vi "MDB Reference.vi"(8 "error in (no error)":errorcluster, 11 "Collaudi T/motori F":bool) -> (0 "error out":errorcluster, 2 "DB rete(F) Locale(T)":bool, 3 "Refnum out":T1)   [LabVIEW 2019]
uses:
  <vilib>/addons/database/Connection.llb/Conn ObjectReference.ctl
  <vilib>/Utility/file.llb/Read From Spreadsheet File (string).vi
  <vilib>/addons/database/Connection.llb/DB Tools Open Connec (String).vi
  Global scelta DB rete o Locale.vi
  <vilib>/addons/database/Connection.llb/DB Tools Open Connec (Path).vi
  <vilib>/addons/database/NI_Database_API.lvlib
panel:
  out "Numeric":i32
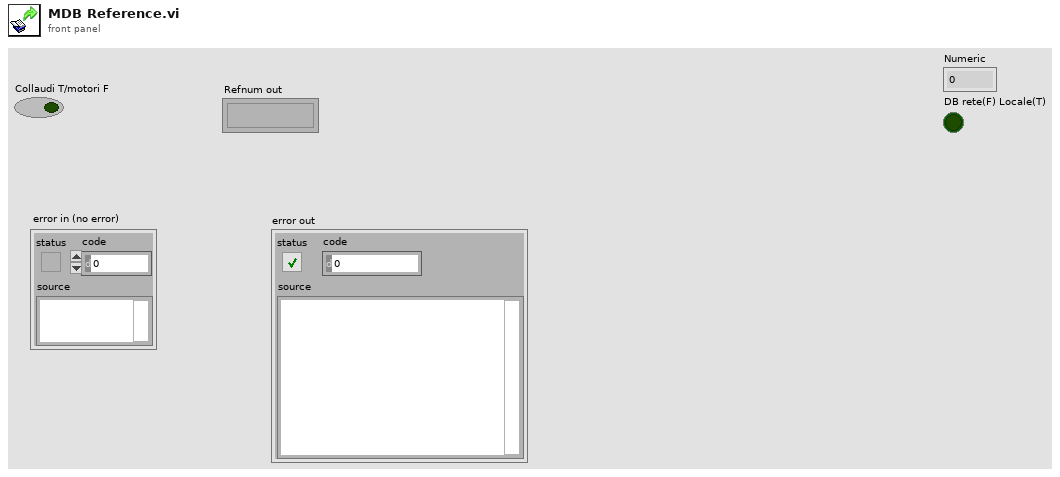
[diagram p1: front panel]
types:
  T1 = typedef "NI_Database_API.lvlib/Conn ObjectReference.ctl" = refnum<k1>
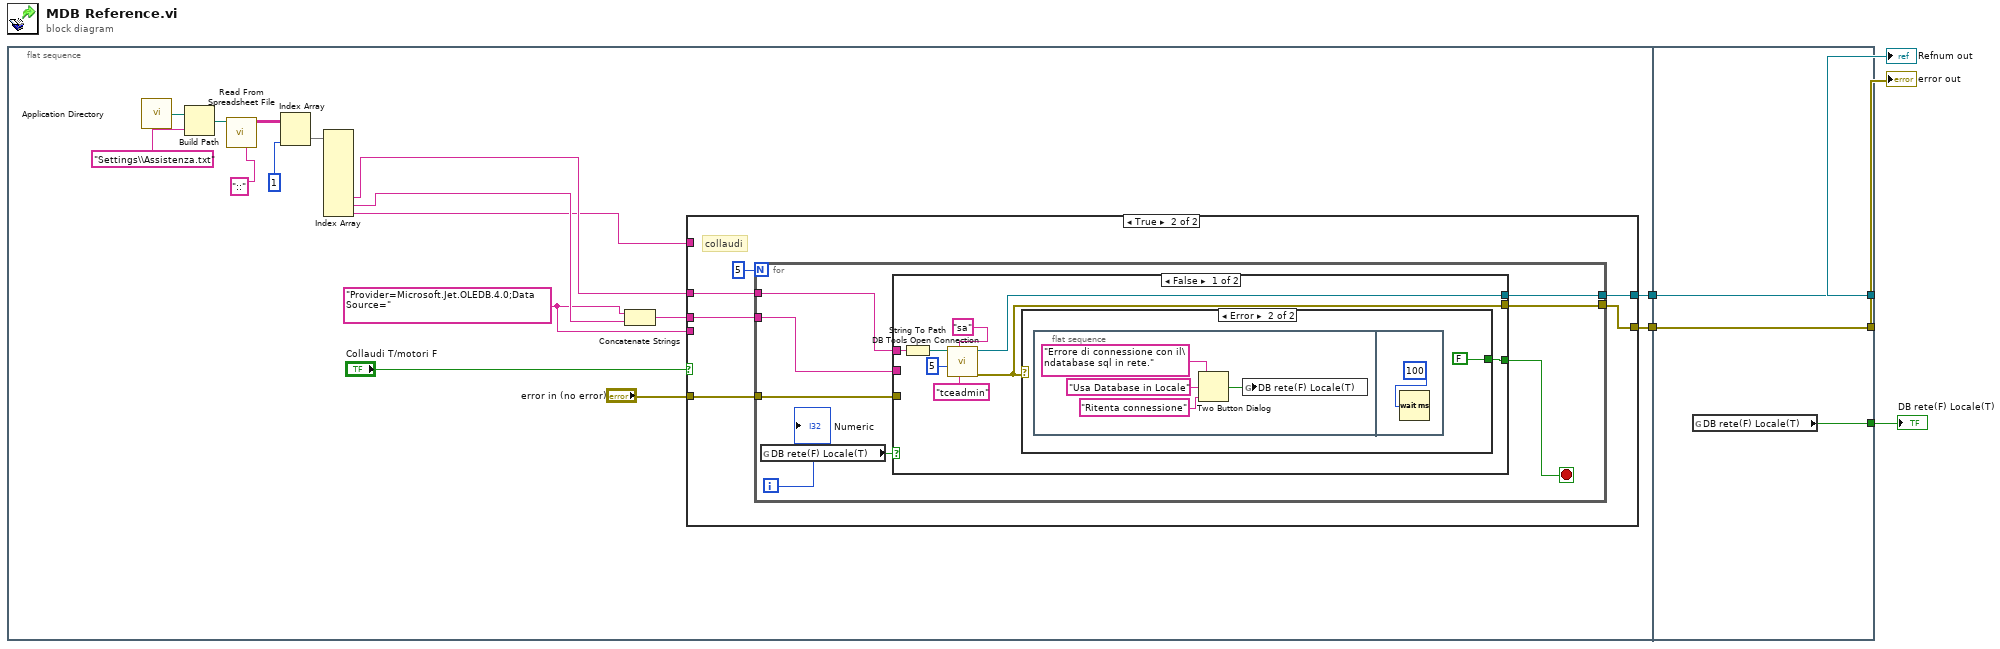
[diagram p0: block diagram]
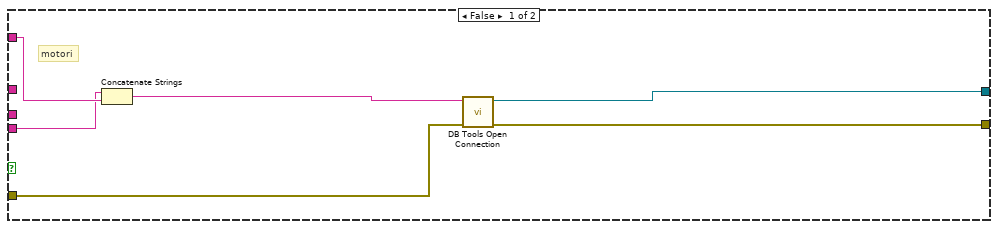
[diagram p2: hidden frame]
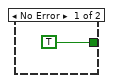
[diagram p3: hidden frame]
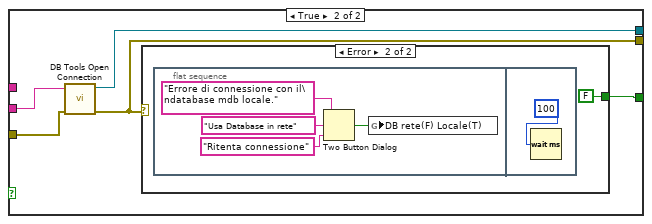
[diagram p4: hidden frame]
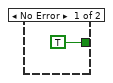
[diagram p5: hidden frame]
diagram:
  n1 = flat-sequence {
    tunnel: [w10] -> w3
    tunnel: [w8] -> w2
    tunnel: [w70] -> w4
    tunnel: [w71] -> w5
    tunnel: w3 -> [w71]
    tunnel: w2 -> [w70]
    tunnel: [w69] -> w1
    frame #0 {
      w6 = "Provider=Microsoft.Jet.OLEDB.4.0;Data Source=" ("userID")
      n2 = call <vilib>:"Application Directory.vi"() -> ("Application Directory"=w21:path)
      n3 = Build Path(base path=w21, name or relative path="Settings\\Assistenza.txt") -> (appended path=w19:path)
      n4 = call-poly <vilib>:"Read From Spreadsheet File.vi"("delimiter (\\t)"="::" ("delimiter (\\t)"), "file path (dialog if empty)"=w19) -> ("all rows"=w18:string[][])  [unwired: 5 in, 4 out]
      n5 = Index Array(array=w18, index (col)=1 ("disabled index (col)")) -> (element=w16:string[])  [unwired: 1 in]
      n6 = Index Array(array=w16) -> (element #7=w13:string, element #8=w12:string, element #9=w9:string)  [unwired: 9 in, 6 out]
      n7 = Concatenate Strings(w6, w12) -> (w11:string)
      n8 = case shown="True" "Collaudi T/motori F" {
        tunnel: w13 -> [_ w33]
        tunnel: w11 -> [_ w32]
        tunnel: [w27 w30] -> w10
        tunnel: w9 -> [w24 _]
        tunnel: [w26 w28] -> w8
        tunnel: "error in (no error)" -> [w25 w29]
        tunnel: w6 -> [w22 _]
        frame False {
          # "motori"
          n9 = Concatenate Strings(w22, w24) -> (w23:string)
          n10 = call-poly <vilib>:"DB Tools Open Connection.vi"("error in (no error)"=w25, "connection information"=w23) -> ("error out"=w26:errorcluster, "connection reference"=w27:T1)  [unwired: 6 in]
        }
        frame True {
          # "collaudi"
          n11 = for {
            N: 5 -> [_]
            tunnel: w33 -> [w41]
            tunnel: w32 -> [w38]
            tunnel: [w37] -> w30
            tunnel: w29 -> [w36]
            tunnel: [w35] -> w28
            i -> [w34]
            stop <- w39 stop-if-true
            n12 = global read "Global scelta DB rete o Locale.vi" "DB rete(F) Locale(T)"() -> (w40:bool)
            n13 = case shown="False" w40 {
              tunnel: w41 -> [w48 _]
              tunnel: [w47 w61] -> w39
              tunnel: w38 -> [_ w60]
              tunnel: [w44 w59] -> w37
              tunnel: w36 -> [_ w58]
              tunnel: [w43 w57] -> w35
              frame False {
                n14 = String To Path(string=w48) -> (path=w49:path)
                n15 = call-poly <vilib>:"DB Tools Open Connection.vi"("password"="tceadmin", "userID"="sa", "connection timeout (15)"=5, "connection information"=w49) -> ("error out"=w43:errorcluster, "connection reference"=w44:T1)  [unwired: 4 in]
                n16 = case shown="Error" w43 {
                  tunnel: [TRUE FALSE] -> w47
                  frame No Error {
                  }
                  frame Error {
                    n17 = flat-sequence {
                      frame #0 {
                        n18 = Two Button Dialog(message="Errore di connessione con il\ndatabase sql in rete.", 1:"Ritenta connessione" ("T button name (\"OK\")"), 2:"Usa Database in Locale" ("T button name (\"OK\")")) -> (T button?=w52:bool)
                        n19 = global write "Global scelta DB rete o Locale.vi" "DB rete(F) Locale(T)"(w52) -> ()
                      }
                      frame #1 {
                        n20 = Wait (ms)(milliseconds to wait=100) -> ()  [unwired: 1 out]
                      }
                    }
                  }
                }
              }
              frame True {
                n21 = call-poly <vilib>:"DB Tools Open Connection.vi"("error in (no error)"=w58, "connection information"=w60) -> ("error out"=w57:errorcluster, "connection reference"=w59:T1)  [unwired: 6 in]
                n22 = case shown="Error" w57 {
                  tunnel: [TRUE FALSE] -> w61
                  frame No Error {
                  }
                  frame Error {
                    n23 = flat-sequence {
                      frame #0 {
                        n24 = Two Button Dialog(message="Errore di connessione con il\ndatabase mdb locale.", 1:"Ritenta connessione" ("T button name (\"OK\")"), 2:"Usa Database in rete" ("T button name (\"OK\")")) -> (T button?=w64:bool)
                        n25 = global write "Global scelta DB rete o Locale.vi" "DB rete(F) Locale(T)"(w64) -> ()
                      }
                      frame #1 {
                        n26 = Wait (ms)(milliseconds to wait=100) -> ()  [unwired: 1 out]
                      }
                    }
                  }
                }
              }
            }
            "Numeric" <- w34
          }
        }
      }
    }
    frame #1 {
      n27 = global read "Global scelta DB rete o Locale.vi" "DB rete(F) Locale(T)"() -> (w69:bool)
    }
  }
  "error out" <- w4
  "Refnum out" <- w5
  "DB rete(F) Locale(T)" <- w1
